vi "TDTSyn-Open Tank.vi"(0 "State In":T1, 11 "error in (no error)":errorcluster) -> (4 "State Out":T1, 15 "error out":errorcluster)   [LabVIEW 2020]
uses:
  TDTSyn-State.ctl
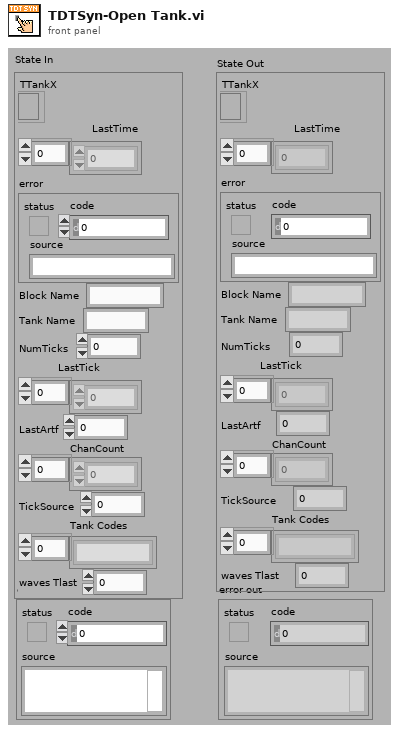
[diagram p1: front panel]
types:
  T1 = typedef "TDTSyn-State.ctl" = cluster{"TTankX":refnum<k7>, "LastTime":dbl[], "error":errorcluster, "Block Name":string, "Tank Name":string, "NumTicks":i32, "LastTick":dbl[], "LastArtf":dbl, "ChanCount":i32[], "TickSource":i32, "Tank Codes":string[], "waves Tlast":dbl}
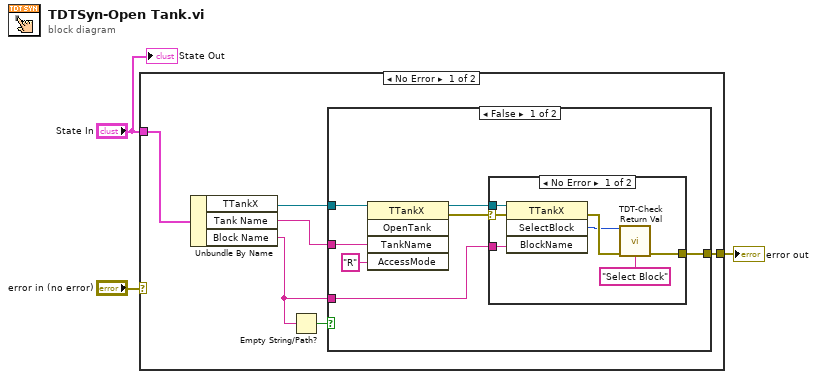
[diagram p0: block diagram]
diagram:
  n1 = case shown="No Error" "error in (no error)" {
    selector: "error in (no error)" -> [_ w25]
    tunnel: [w9 w25] -> w2
    tunnel: "State In" -> [w6 _]
    frame No Error {
      n2 = Unbundle By Name(w6) -> ("TTankX"=w7:refnum<k7>, "Tank Name"=w8:string, "Block Name"=w4:string)
      n3 = Empty String/Path?(string/path=w4) -> (empty?=w5:bool)
      n4 = case shown="False" w5 {
        tunnel: [w16 _] -> w9
        tunnel: w8 -> [w11 _]
        tunnel: w7 -> [w15 _]
        tunnel: w4 -> [w10 _]
        frame False {
          n5 = invoke class="TTankX" method="OpenTank"(reference=w15, "TankName"=w11, "AccessMode"="R") -> (reference out=w14:refnum<k7>, error out=w12:errorcluster)  [unwired: 2 in, 3 out]
          n6 = case shown="No Error" w12 {
            selector: w12 -> [w18 w24]
            tunnel: [w22 w24] -> w16
            tunnel: w14 -> [w21 _]
            tunnel: w10 -> [w17 _]
            frame No Error {
              n7 = invoke class="TTankX" method="SelectBlock"(reference=w21, error in=w18, "BlockName"=w17) -> (error out=w20:errorcluster, "SelectBlock"=w19:i32)  [unwired: 1 in, 2 out]
              n8 = call "TDT-Check Return Val.vi"("Return Val"=w19, "error in (no error)"=w20, "source"="Select Block" ("Message")) -> ("error out"=w22:errorcluster)  [unwired: 12 in]
            }
            frame Error {
            }
          }
        }
        frame True {
        }
      }
    }
    frame Error {
    }
  }
  "error out" <- w2
  "State Out" <- "State In"
